vi "Path_generation_isle.vi"(0 "Projektname":string, 3 "Basis-Pfad":path, 5 "error in (no error)":errorcluster caption="Fehler (Eingang, kein Fehler)", 7 "Pfad erstellen ? [T]":bool, 9 "Revison":i32=1) -> (11 "Größe des Datenträgers (GB)":ext format="%#.2f", 13 "Freier Speicher (GB)":ext, 15 "Projektname inkl. Revisionsnr.":string, 16 "Erstellter Pfad":path, 19 "error out":errorcluster={"status"=TRUE, "code"=10, "source"=""} caption="Fehler (Ausgang)")   [LabVIEW 2014]
doc: "Dieses VI erstellt in Abhängigkeit des Projektnamens einen Pfad. \n\nIst dieser Pfad schon vorhanden wird ein fortlaufender Revisionsindex RXXX angehängt.\nDer erstellte Pfad beinhaltet außerdem das Erstellungsdatum.\n\nProjektname_JJJJ-MM-DD_RXXX"
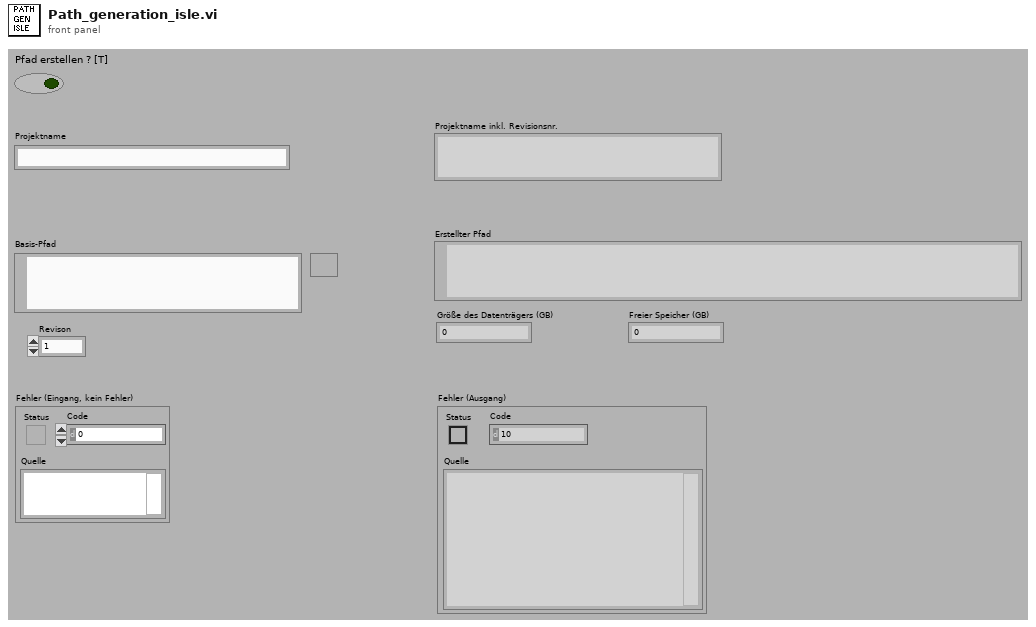
[diagram p1: front panel]
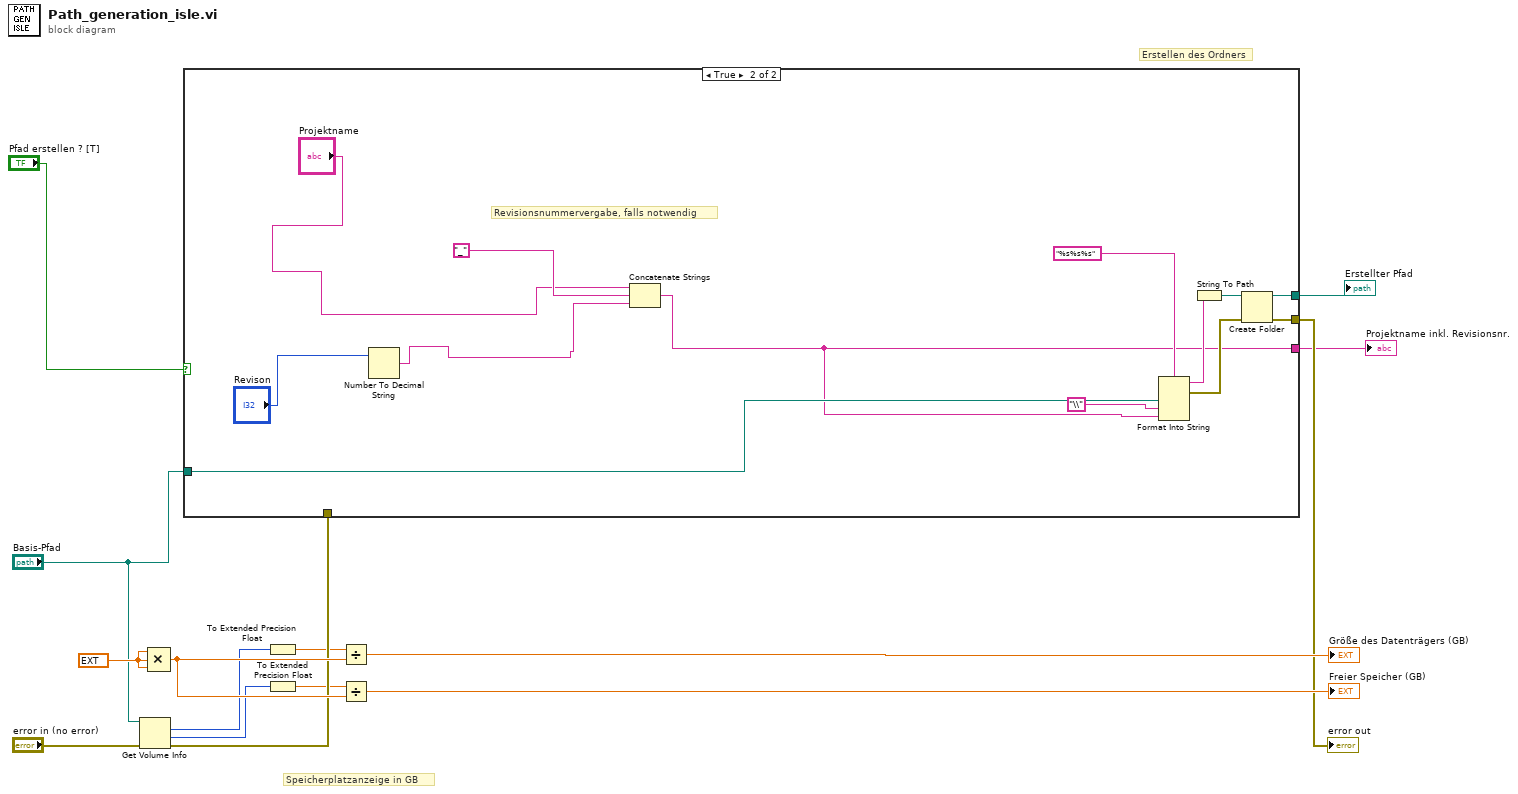
[diagram p0: block diagram]
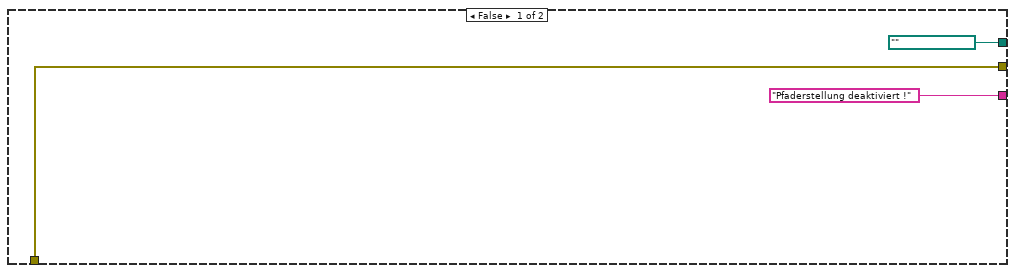
[diagram p2: hidden frame]
diagram:
  w11 = ext 1024.0
  # "Erstellen des Ordners"
  # "Speicherplatzanzeige in GB"
  n1 = Get Volume Info(8:"error in (no error)", 11:"Basis-Pfad") -> (0:w7:errorcluster, 1:w3:i64, 2:w5:i64)  [unwired: 3 out]
  n2 = Compound Arithmetic op=MULTIPLY(w11, w11, w11) -> (w10:ext)
  n3 = case shown="True" "Pfad erstellen ? [T]" {
    tunnel: [path "" ("created path") w30] -> w15
    tunnel: "Basis-Pfad" -> [_ w27]
    tunnel: [w18 w29] -> w8
    tunnel: w7 -> [w18 _]
    tunnel: ["Pfaderstellung deaktiviert !" w20] -> w2
    frame False {
    }
    frame True {
      # "Revisionsnummervergabe, falls notwendig"
      n4 = Number To Decimal String(number="Revison") -> (decimal integer string=w22:string)  [unwired: 1 in]
      n5 = Concatenate Strings("Projektname", "_" ("String"), w22) -> (w20:string)
      n6 = Format Into String(format string="%s%s%s" ("Format-String"), w27, "\\" ("Eingang 2"), w20) -> (resulting string=w26:string, error out=w25:errorcluster)  [unwired: 2 in]
      n7 = String To Path(string=w26) -> (path=w31:path)
      n8 = Create Folder(path (use dialog)=w31, error in=w25) -> (created path=w30:path, error out=w29:errorcluster)  [unwired: 1 in, 1 out]
    }
  }
  "error out" <- w8
  "Erstellter Pfad" <- w15
  "Projektname inkl. Revisionsnr." <- w2
  n9 = To Extended Precision Float(1:w5) -> (0:w6:ext)
  n10 = To Extended Precision Float(1:w3) -> (0:w4:ext)
  n11 = Divide(x=w6, y=w10) -> (x/y=→"Größe des Datenträgers (GB)":ext)
  n12 = Divide(x=w4, y=w10) -> (x/y=→"Freier Speicher (GB)":ext)
